vi "Global_MdlMgmt.vi"() -> ()   [LabVIEW 2016]
doc: "-----------------------------------------------------------------------------------------------------------------------\nCopyright <2019> <The University of Tennessee at Knoxville and the University of Tennessee Research Foundation>\nThis software is released under BSD-3 \nhttps://opensource.org/licenses/BSD-3-Clause \nAdditional license options available at https://utrf.tennessee.edu/industry/sample-agreements/\n-----------------------------------------------------------------------------------------------------------------------"
panel:
  in  "State_est BESS location":dbl[](array[numeric])
  in  "Equally Metrix":dbl[][](array[numeric])
  in  "Grid Interface":dbl[](array[numeric])
  in  "To Topology Identification":dbl[][](array[numeric])
  in  "Microgrid Topology Overall":dbl[][](array[numeric])
  in  "Slack_bus":dbl[](array[numeric])
  in  "node_relationship_StaEst":dbl[][](array[numeric])
  in  "Switch number":dbl
  in  "PV inverter current limit":dbl
  in  "PV number":dbl
  in  "PQ discharge max SoC":dbl
  in  "PQ recharge min SoC":dbl
  in  "PQ cycle time":dbl
  in  "PQ BESS location":dbl[](array[numeric])
  in  "Load history active/reacitve power":dbl[][](array[numeric])
  in  "BESS inverter current limit":dbl
  in  "BESS number":dbl
  in  "BESS max Freq":dbl
  in  "BESS min Freq":dbl
  in  "BESS max Vol":dbl
  in  "BESS min Vol":dbl
  in  "BESS max SoC":dbl
  in  "BESS Capacity":dbl
  in  "BESS Power limit":dbl
  in  "BESS min SoC":dbl
  in  "PV location":dbl[](array[numeric])
  in  "BESS location":dbl[](array[numeric])
  in  "Grid connect interface location":dbl[](array[numeric])
  in  "Microgrid Topology":dbl[][](array[numeric])
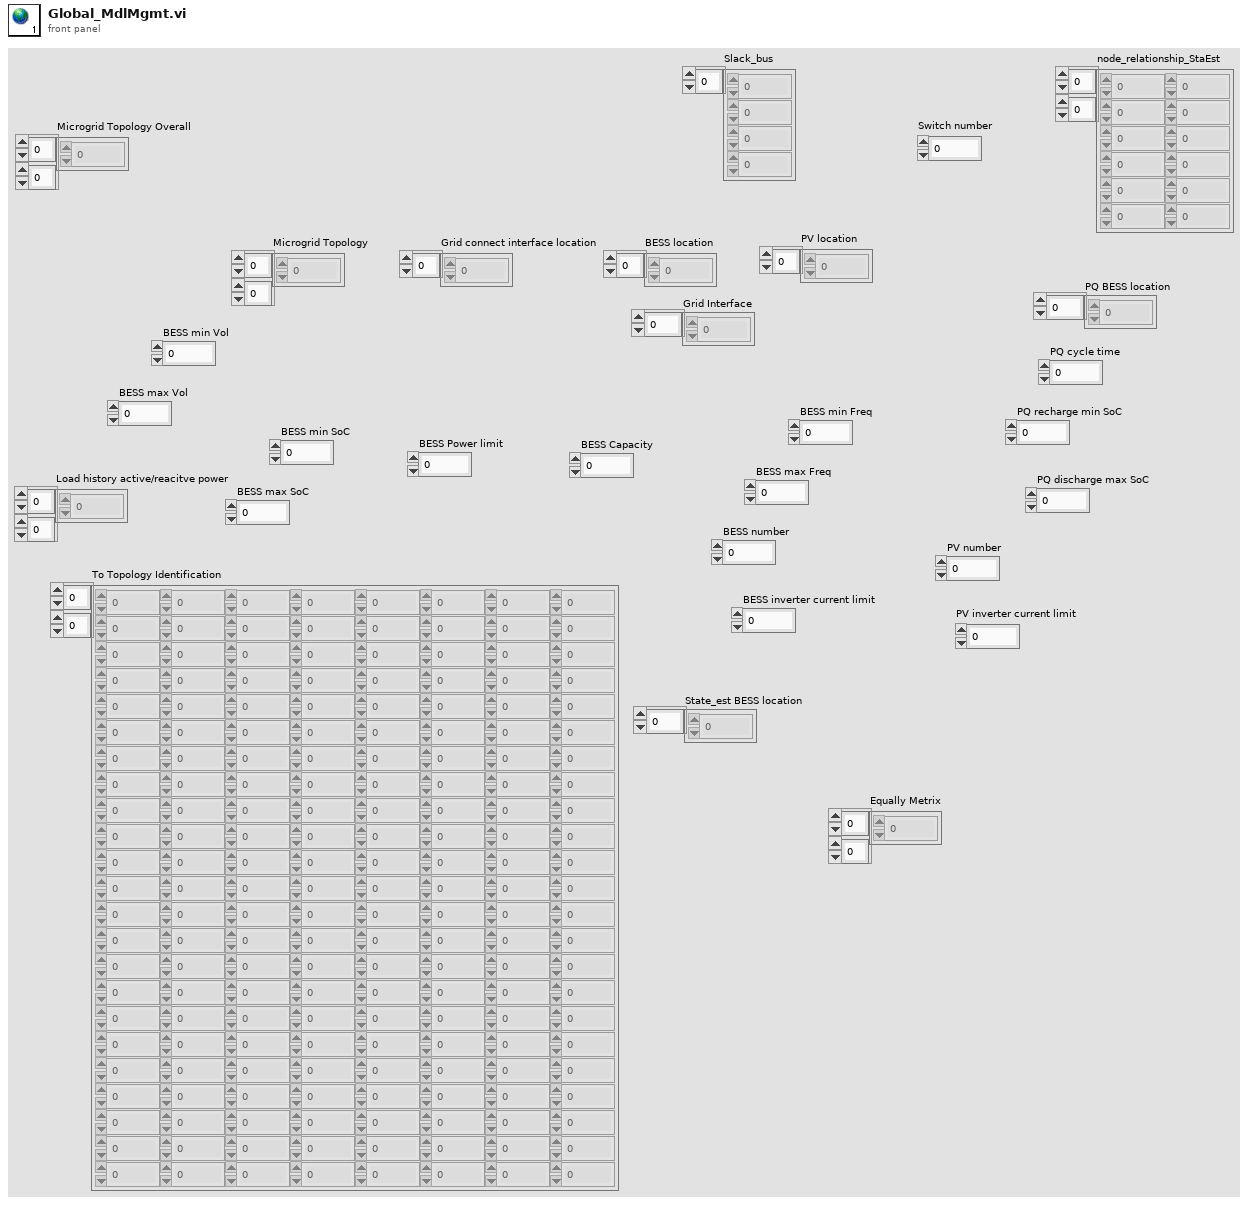
[diagram p1: front panel]
diagram:
